vi "Test_Listen.vi"(8 "error in":errorcluster, 11 "Port":string="COM13") -> (0 "error out":errorcluster, 2 "Read":T1)   [LabVIEW 2016, in "Serial_G.lvlib"]
doc: "Tests a cmd"
uses:
  Serial_G.lvlib
  Controls/Cmd_Rx.ctl
  Controls/PortConfig.ctl
panel:
  in  "Delay_ms":u32=250
  in  "Exit":bool
  out "Port?":bool
  # "Serial Communication Driver - (Rx)"
  # "Response                                                            Exec time   Timeout?"
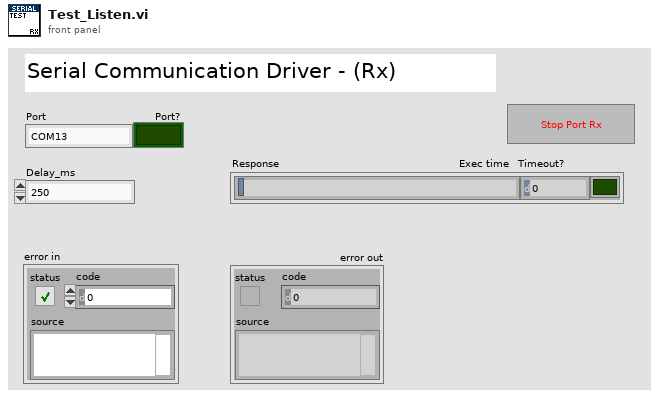
[diagram p1: front panel]
types:
  T1 = typedef "Serial_G.lvlib/Cmd_Rx.ctl" = cluster{"Read":string, "ExecTime (ms)":i32, "Timeout?":bool}
  T2 = typedef "Serial_G.lvlib/PortConfig.ctl" = cluster{"Baud rate":u32, "Parity":enum16{"None", "Odd", "Even", "Mark", "Space"}, "Data bits":u16, "Stop bits":u16, "Flow control":u16}
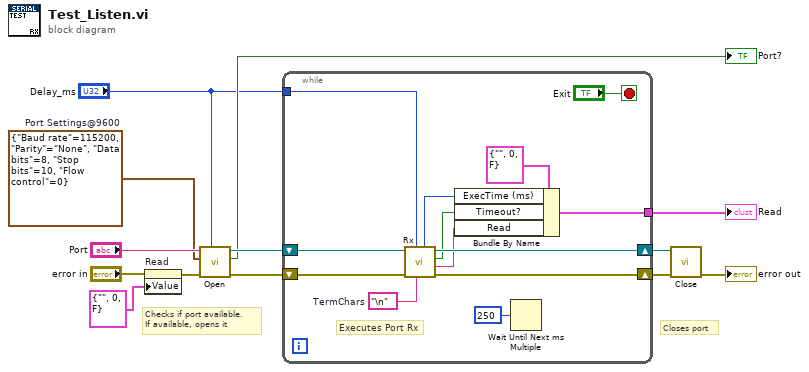
[diagram p0: block diagram]
diagram:
  w2 = T2 {"Baud rate"=115200, "Parity"=enum."None", "Data bits"=8, "Stop bits"=10, "Flow control"=0}  # Port Settings@9600
  # "Closes port"
  # "Checks if port available.\nIf available, opens it"
  n1 = property on="Read" class="Clust (strict)"(error in="error in", "Value"=T1 {"Read"="", "ExecTime (ms)"=0, "Timeout?"=FALSE} ("Read")) -> (error out=w6:errorcluster)  [unwired: 1 in, 1 out]
  n2 = call "Open.vi"("Timeout (3000)"="Delay_ms", "error in"=w6, "ConfigPort (9600,0,8,1)"=w2, "Port(Alias)"="Port") -> ("error out"=w13:errorcluster, "PortFound?"=→"Port?":bool, "VISA out"=w12:refnum<visa-resource-name>)  [unwired: 4 in, 1 out]
  n3 = while {
    tunnel: [w21] -> w3
    shift-right: [w23] -> w9
    shift-left: w13 -> [w26]
    shift-right: [w24] -> w11
    shift-left: w12 -> [w25]
    tunnel: "Delay_ms" -> [w14]
    stop <- "Exit" stop-if-true
    w17 = "\n"  # TermChars
    # "Executes Port Rx"
    n4 = call "Rx.vi"("Wait for? (\\r\\n)"=w17, "Timeout_ms (3000)"=w14, "error in"=w26, "VISA in"=w25) -> ("error out"=w23:errorcluster, "Response"=w20:string, "Timeout?"=w19:bool, "VISA out"=w24:refnum<visa-resource-name>, "ExecTime(ms)"=w18:i32)  [unwired: 3 in]
    n5 = Bundle By Name(cluster=T1 {"Read"="", "ExecTime (ms)"=0, "Timeout?"=FALSE} ("Read"), "ExecTime (ms)"=w18, "Timeout?"=w19, "Read"=w20) -> (w21:T1)
    n6 = Wait Until Next ms Multiple(millisecond multiple=u32 250) -> ()  [unwired: 1 out]
  }
  "Read" <- w3
  n7 = call "Close.vi"("error in"=w9, "VISA in"=w11) -> ("error out"=→"error out":errorcluster)  [unwired: 9 in]
